vi "Audio.Find FFT Peaks.vi"() -> ()   [LabVIEW 2018]
uses:
  <vilib>/Analysis/5stat.llb/RMS (DBL).vi
  <vilib>/Analysis/NI_AALPro.lvlib
panel:
  out "max value":dbl
  out "RMS":dbl
  in  "Max":dbl=1100.0
  in  "Min":dbl=900.0
  in  "FFT Left":cluster{"f0":dbl, "df":dbl, "magnitude":dbl[]}(graph)
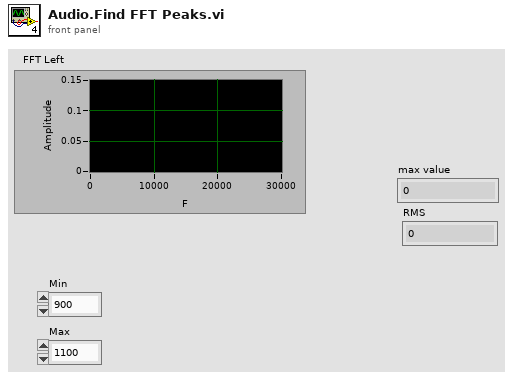
[diagram p1: front panel]
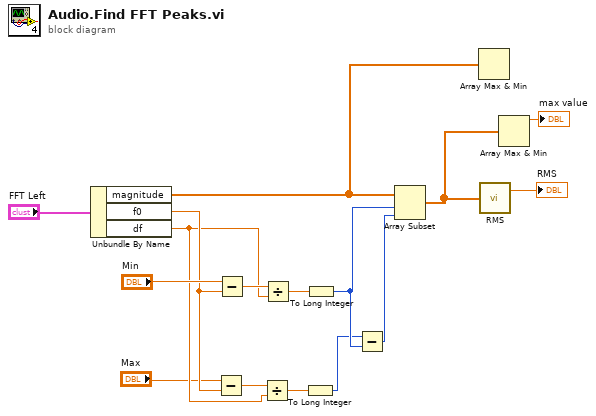
[diagram p0: block diagram]
diagram:
  n1 = Unbundle By Name("FFT Left") -> ("magnitude"=w2:dbl[], "f0"=w11:dbl, "df"=w10:dbl)
  n2 = Subtract(x="Max", y=w11) -> (x-y=w12:dbl)
  n3 = Subtract(x="Min", y=w11) -> (x-y=w15:dbl)
  n4 = Divide(x=w12, y=w10) -> (x/y=w13:dbl)
  n5 = Divide(x=w15, y=w10) -> (x/y=w14:dbl)
  n6 = To Long Integer(number=w13) -> (32bit integer=w7:i32)
  n7 = To Long Integer(number=w14) -> (32bit integer=w8:i32)
  n8 = Subtract(x=w7, y=w8) -> (x-y=w6:i32)
  n9 = Array Subset(array=w2, index=w8, length=w6) -> (w4:dbl[])
  n10 = Array Max & Min(array=w2) -> ()  [unwired: 4 out]
  n11 = call-poly <vilib>:"RMS.vi"("X"=w4) -> ("rms value"=→"RMS":dbl)  [unwired: 1 out]
  n12 = Array Max & Min(array=w4) -> (max value=→"max value":dbl)  [unwired: 3 out]
